vi "Test Write Structs.vi"(11 "TwinCAT ADS in":refnum<class "TwinCAT ADS.lvclass">) -> (3 "TwinCAT ADS out":refnum<class "TwinCAT ADS.lvclass">)   [LabVIEW 2018]
uses:
  TwinCAT ADS Class/TwinCAT ADS.lvclass
  Controls/ST_Simple.ctl
  Controls/ST_Packed.ctl
  Controls/ST_Complex.ctl
  Controls/Enum.ctl
  Controls/FB_Simple.ctl
  23fdef96-acda-4c8c-ba2d-722c4e2ed0c7.vi
  3ed625e2-61d1-494e-80f8-eda327ae6200.vi
  f38583b2-ec11-48cf-baad-4002a53f8002.vi
  81473f10-2869-4eaa-9cd5-fba83cff517c.vi
  67abcce4-d906-4956-a77e-4a47c9dde040.vi
  903064a7-6281-4536-8159-57f8726da337.vi
  TwinCAT ADS Class/VIs/Data/Read.vi
  <vilib>/addons/_JKI Toolkits/Caraya/classes/Assert/Assert True.vi
  <vilib>/addons/_JKI Toolkits/Caraya/classes/Test/Test.lvclass
  <vilib>/addons/_JKI Toolkits/Caraya/classes/Assert/Assert.lvclass
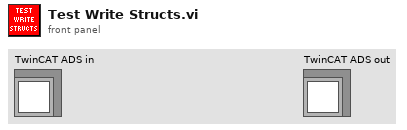
[diagram p1: front panel]
types:
  T1 = typedef "ST_Complex.ctl" = cluster{"bMember":bool, "eMember":T2, "stSimpleMember":T3, "stPackedMember":T4, "FB_Simple":T5, "arrfMember":dbl[]}
  T2 = typedef "Enum.ctl" = enum16{"Member 0", "Member 1", "Member 2"}
  T3 = typedef "ST_Simple.ctl" = cluster{"bMember":bool, "dtMember":timestamp, "nMember":i32}
  T4 = typedef "ST_Packed.ctl" = cluster{"bMember":bool, "dtMember":timestamp, "fMember":dbl}
  T5 = typedef "FB_Simple.ctl" = cluster{"_bMember":bool, "_nMember":i32, "_sMember":string}
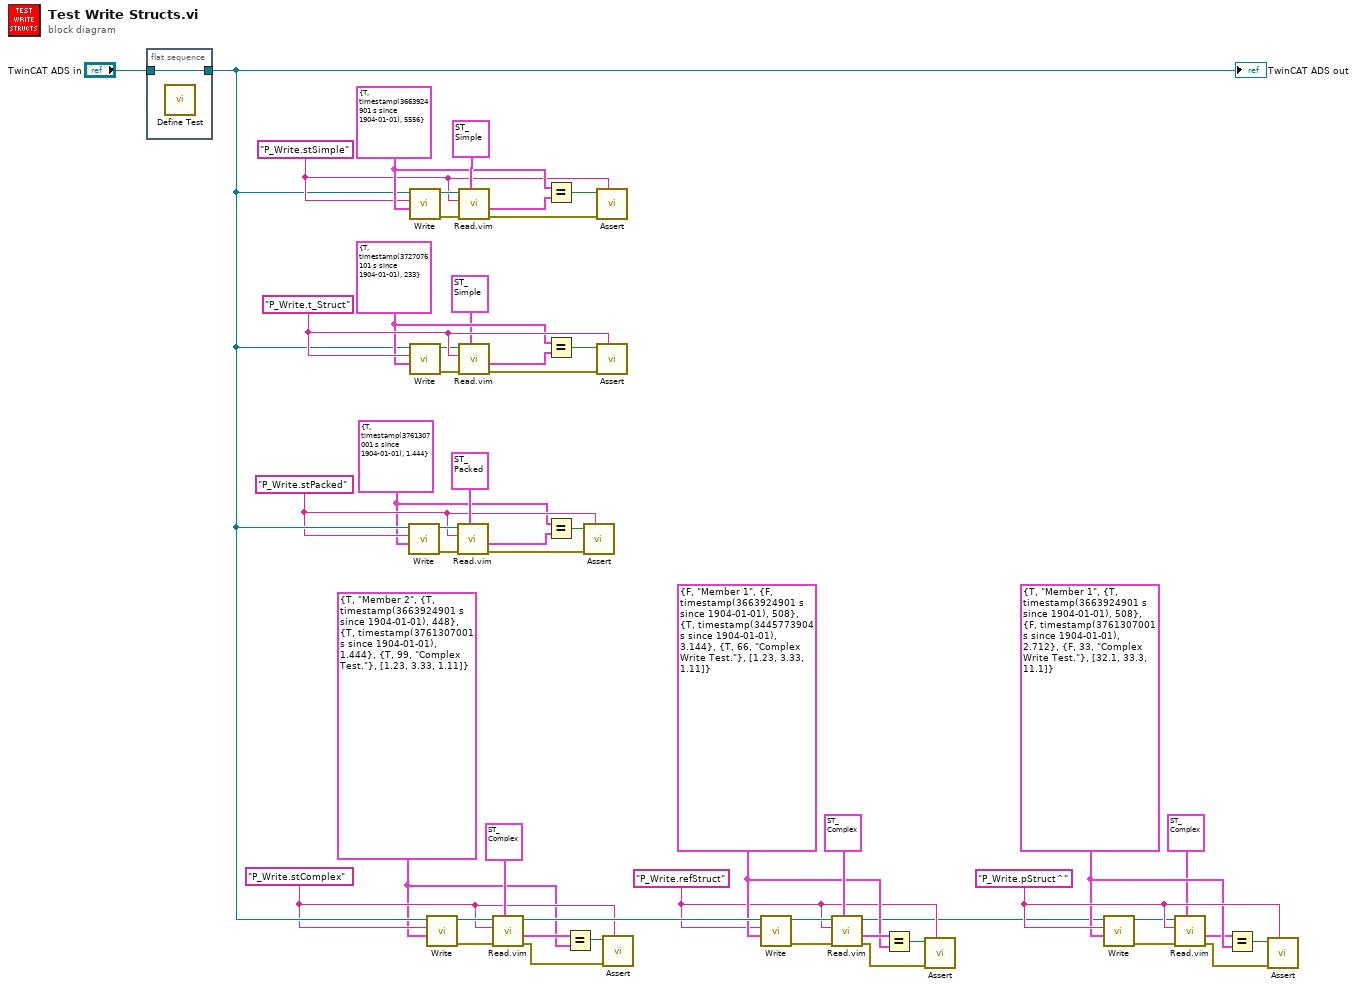
[diagram p0: block diagram]
diagram:
  w8 = T1 {"bMember"=TRUE, "eMember"=enum."Member 1", "stSimpleMember"={"bMember"=TRUE, "dtMember"=timestamp(3663924901 s since 1904-01-01), "nMember"=508}, "stPackedMember"={"bMember"=FALSE, "dtMember"=timestamp(3761307001 s since 1904-01-01), "fMember"=2.712}, "FB_Simple"={"_bMember"=FALSE, "_nMember"=33, "_sMember"="Complex Write Test."}, "arrfMember"=[32.1, 33.3, 11.1]} ("ST_Complex")
  w9 = "P_Write.pStruct^" ("Symbol Name")
  w11 = T1 {"bMember"=FALSE, "eMember"=enum."Member 1", "stSimpleMember"={"bMember"=FALSE, "dtMember"=timestamp(3663924901 s since 1904-01-01), "nMember"=508}, "stPackedMember"={"bMember"=TRUE, "dtMember"=timestamp(3445773904 s since 1904-01-01), "fMember"=3.144}, "FB_Simple"={"_bMember"=TRUE, "_nMember"=66, "_sMember"="Complex Write Test."}, "arrfMember"=[1.23, 3.33, 1.11]} ("ST_Complex")
  w16 = T1 {"bMember"=TRUE, "eMember"=enum."Member 2", "stSimpleMember"={"bMember"=TRUE, "dtMember"=timestamp(3663924901 s since 1904-01-01), "nMember"=448}, "stPackedMember"={"bMember"=TRUE, "dtMember"=timestamp(3761307001 s since 1904-01-01), "fMember"=1.444}, "FB_Simple"={"_bMember"=TRUE, "_nMember"=99, "_sMember"="Complex Test."}, "arrfMember"=[1.23, 3.33, 1.11]} ("ST_Complex")
  w22 = T4 {"bMember"=TRUE, "dtMember"=timestamp(3761307001 s since 1904-01-01), "fMember"=1.444} ("ST_Packed")
  w33 = T3 {"bMember"=TRUE, "dtMember"=timestamp(3727076101 s since 1904-01-01), "nMember"=233} ("ST_Simple")
  w36 = "P_Write.t_Struct" ("Symbol Name")
  w40 = T3 {"bMember"=TRUE, "dtMember"=timestamp(3663924901 s since 1904-01-01), "nMember"=5556} ("ST_Simple")
  w10 = "P_Write.refStruct" ("Symbol Name")
  w19 = "P_Write.stComplex" ("Symbol Name")
  w24 = "P_Write.stPacked" ("Symbol Name")
  w37 = "P_Write.stSimple" ("Symbol Name")
  n1 = flat-sequence {
    tunnel: "TwinCAT ADS in" -> [w53]
    tunnel: [w53] -> w28
    frame #0 {
      n2 = call <vilib>:"Define Test.vi"() -> ()  [unwired: 10 in, 2 out]
    }
  }
  n3 = call "Write.vi"("Value"=w22, "Symbol Name"=w24, "TwinCAT ADS in"=w28) -> ("error out"=w49:errorcluster, "TwinCAT ADS out"=w48:refnum<class "TwinCAT ADS.lvclass">)  [unwired: 7 in]
  n4 = call "Write.vi"("Value"=w40, "Symbol Name"=w37, "TwinCAT ADS in"=w28) -> ("error out"=w50:errorcluster, "TwinCAT ADS out"=w51:refnum<class "TwinCAT ADS.lvclass">)  [unwired: 7 in]
  n5 = call "Write.vi"("Value"=w33, "Symbol Name"=w36, "TwinCAT ADS in"=w28) -> ("error out"=w30:errorcluster, "TwinCAT ADS out"=w29:refnum<class "TwinCAT ADS.lvclass">)  [unwired: 7 in]
  n6 = call "Write.vi"("Value"=w16, "Symbol Name"=w19, "TwinCAT ADS in"=w28) -> ("error out"=w46:errorcluster, "TwinCAT ADS out"=w47:refnum<class "TwinCAT ADS.lvclass">)  [unwired: 7 in]
  n7 = call "Read.vim"("Type"=T4 {"bMember"=FALSE, "dtMember"=timestamp(0 s since 1904-01-01), "fMember"=0.0} ("ST_Packed"), "error in (no error)"=w49, "Symbol Name"=w24, "TwinCAT ADS in"=w48) -> ("error out"=w26:errorcluster, "Value"=w23:T4)  [unwired: 5 in, 1 out]
  n8 = call "Read.vim"("Type"=T3 {"bMember"=FALSE, "dtMember"=timestamp(0 s since 1904-01-01), "nMember"=0} ("ST_Simple"), "error in (no error)"=w50, "Symbol Name"=w37, "TwinCAT ADS in"=w51) -> ("error out"=w41:errorcluster, "Value"=w39:T3)  [unwired: 5 in, 1 out]
  n9 = call "Read.vim"("Type"=T3 {"bMember"=FALSE, "dtMember"=timestamp(0 s since 1904-01-01), "nMember"=0} ("ST_Simple"), "error in (no error)"=w30, "Symbol Name"=w36, "TwinCAT ADS in"=w29) -> ("error out"=w32:errorcluster, "Value"=w34:T3)  [unwired: 5 in, 1 out]
  n10 = call "Read.vim"("Type"=T1 {"bMember"=FALSE, "eMember"=enum."Member 0", "stSimpleMember"={"bMember"=FALSE, "dtMember"=timestamp(0 s since 1904-01-01), "nMember"=0}, "stPackedMember"={"bMember"=FALSE, "dtMember"=timestamp(0 s since 1904-01-01), "fMember"=0.0}, "FB_Simple"={"_bMember"=FALSE, "_nMember"=0, "_sMember"=""}, "arrfMember"=[]} ("ST_Complex"), "error in (no error)"=w46, "Symbol Name"=w19, "TwinCAT ADS in"=w47) -> ("error out"=w20:errorcluster, "Value"=w17:T1, "TwinCAT ADS out"=w43:refnum<class "TwinCAT ADS.lvclass">)  [unwired: 5 in]
  n11 = Equal?(x=w40, y=w39) -> (x = y?=w38:bool)
  n12 = Equal?(x=w33, y=w34) -> (x = y?=w35:bool)
  n13 = Equal?(x=w22, y=w23) -> (x = y?=w25:bool)
  n14 = Equal?(x=w17, y=w16) -> (x = y?=w18:bool)
  n15 = call-poly <vilib>:"Assert.vi"("Label"=w24, "error in (no error)"=w26, "True?"=w25) -> ()  [unwired: 7 in, 2 out]
  n16 = call-poly <vilib>:"Assert.vi"("Label"=w37, "error in (no error)"=w41, "True?"=w38) -> ()  [unwired: 7 in, 2 out]
  n17 = call-poly <vilib>:"Assert.vi"("Label"=w36, "error in (no error)"=w32, "True?"=w35) -> ()  [unwired: 7 in, 2 out]
  n18 = call-poly <vilib>:"Assert.vi"("Label"=w19, "error in (no error)"=w20, "True?"=w18) -> ()  [unwired: 7 in, 2 out]
  n19 = call "Write.vi"("Value"=w11, "Symbol Name"=w10, "TwinCAT ADS in"=w43) -> ("error out"=w44:errorcluster, "TwinCAT ADS out"=w45:refnum<class "TwinCAT ADS.lvclass">)  [unwired: 7 in]
  n20 = call "Read.vim"("Type"=T1 {"bMember"=FALSE, "eMember"=enum."Member 0", "stSimpleMember"={"bMember"=FALSE, "dtMember"=timestamp(0 s since 1904-01-01), "nMember"=0}, "stPackedMember"={"bMember"=FALSE, "dtMember"=timestamp(0 s since 1904-01-01), "fMember"=0.0}, "FB_Simple"={"_bMember"=FALSE, "_nMember"=0, "_sMember"=""}, "arrfMember"=[]} ("ST_Complex"), "error in (no error)"=w44, "Symbol Name"=w10, "TwinCAT ADS in"=w45) -> ("error out"=w13:errorcluster, "Value"=w14:T1, "TwinCAT ADS out"=w1:refnum<class "TwinCAT ADS.lvclass">)  [unwired: 5 in]
  n21 = Equal?(x=w14, y=w11) -> (x = y?=w12:bool)
  n22 = call-poly <vilib>:"Assert.vi"("Label"=w10, "error in (no error)"=w13, "True?"=w12) -> ()  [unwired: 7 in, 2 out]
  n23 = call "Write.vi"("Value"=w8, "Symbol Name"=w9, "TwinCAT ADS in"=w1) -> ("error out"=w3:errorcluster, "TwinCAT ADS out"=w2:refnum<class "TwinCAT ADS.lvclass">)  [unwired: 7 in]
  n24 = call "Read.vim"("Type"=T1 {"bMember"=FALSE, "eMember"=enum."Member 0", "stSimpleMember"={"bMember"=FALSE, "dtMember"=timestamp(0 s since 1904-01-01), "nMember"=0}, "stPackedMember"={"bMember"=FALSE, "dtMember"=timestamp(0 s since 1904-01-01), "fMember"=0.0}, "FB_Simple"={"_bMember"=FALSE, "_nMember"=0, "_sMember"=""}, "arrfMember"=[]} ("ST_Complex"), "error in (no error)"=w3, "Symbol Name"=w9, "TwinCAT ADS in"=w2) -> ("error out"=w6:errorcluster, "Value"=w5:T1)  [unwired: 5 in, 1 out]
  n25 = Equal?(x=w5, y=w8) -> (x = y?=w7:bool)
  n26 = call-poly <vilib>:"Assert.vi"("Label"=w9, "error in (no error)"=w6, "True?"=w7) -> ()  [unwired: 7 in, 2 out]
  "TwinCAT ADS out" <- w28
